vi "Status mit Kalibier Info aktualisieren.vi"(7 "show Status even if no Error":bool, 8 "error in (no error)":errorcluster caption="Fehler (Eingang, kein Fehler)", 10 "Sprachliste":string[][](array[string]), 11 "Kalibrier Info-Cluster in":T1) -> (0 "error out":errorcluster caption="Fehler (Ausgang)", 3 "Status out":string)   [LabVIEW 2020, in "Linearisierung v2.lvlib" / "SpanEinstellungen.lvlib"]
uses:
  SpanEinstellungen.lvlib
  Kalibrier Info Cluster.ctl
  Gasteiler/Aktion FGV Daten Abholung uebergebenctl.ctl
  Gasteiler/Gasteiler.lvlib
  Allgemein/allgemeine Sub-VIs.lvlib
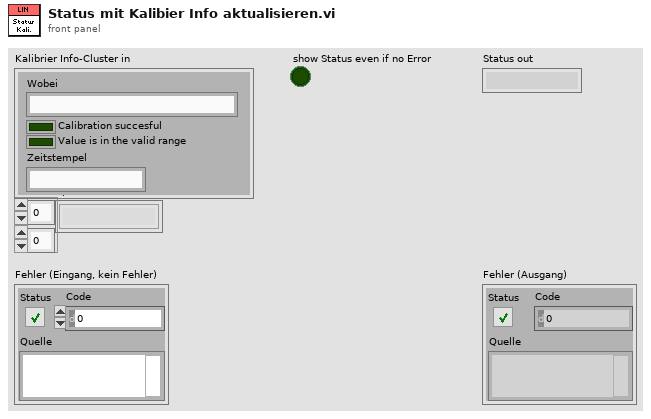
[diagram p1: front panel]
types:
  T1 = typedef "Linearisierung v2.lvlib/SpanEinstellungen.lvlib/Kalibrier Info Cluster.ctl" = cluster{"Wobei":string, "Calibration succesful":bool, "Value is in the valid range":bool, "Zeitstempel":string}
  T2 = typedef "Linearisierung v2.lvlib/Gasteiler.lvlib/Aktion FGV Daten Abholung uebergebenctl.ctl" = enum16{"lesen", "schreiben", "Anzeigebit löschen", "Status hinzufügen"}
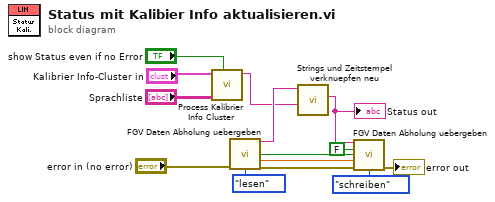
[diagram p0: block diagram]
diagram:
  n1 = call "Process Kalibrier Info Cluster.vi"("show Status even if no Error"="show Status even if no Error", "Sprachliste"="Sprachliste", "Kalibrier Info-Cluster in"="Kalibrier Info-Cluster in") -> ("String"=w4:string)  [unwired: 7 in, 1 out]
  n2 = call "FGV Daten Abholung uebergeben.vi"("error in (no error)"="error in (no error)", "Aktion"=Aktion_FGV_Daten_Abholung_uebergebenctl."lesen") -> ("Zustand"=w9:string, "Beendet"=w10:bool, "Restlaufzeit out"=w11:sgl, "error out"=w12:errorcluster)  [unwired: 9 in, 1 out]
  n3 = call "Strings und Zeitstempel verknuepfen neu.vi"("String 1 hinzufügen"=w4, "Eingangs String"=w9) -> ("Verknüpfter String"=w8:string)  [unwired: 9 in]
  "Status out" <- w8
  n4 = call "FGV Daten Abholung uebergeben.vi"("Zustand"=w8, "Anzeige aktualisieren"=FALSE, "Beendet"=w10, "Restlaufzeit"=w11, "error in (no error)"=w12, "Aktion"=Aktion_FGV_Daten_Abholung_uebergebenctl."schreiben") -> ("error out"=→"error out":errorcluster)  [unwired: 5 in, 4 out]
